vi "Display Fonts Manager.vi"(4 "Error In":errorcluster) -> (0 "Error Out":errorcluster)   [LabVIEW 2020, in "Display Properties Manager.lvlib"]
uses:
  Display Properties Manager.lvlib
  Display Properties.lvclass
  Config Data/Config Data.lvclass
  toolbox/Error Reporting and Storage/Error Reporting and Storage.lvlib
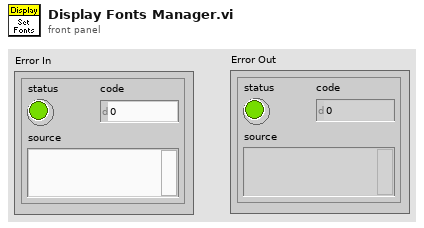
[diagram p1: front panel]
types:
  T1 = typedef "Display Properties Manager.lvlib/Font Parameters.ctl" = cluster{"Font Name":string, "Font Size":u32, "Component to Set":T2}
  T2 = typedef "Display Properties Manager.lvlib/Control Component to Set.ctl" = enum16{"Label", "Caption", "Contents"}
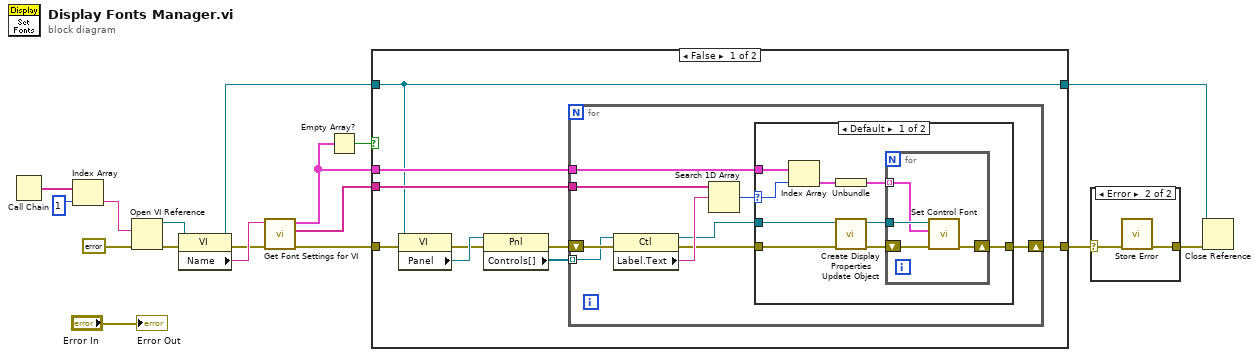
[diagram p0: block diagram]
diagram:
  n1 = Call Chain() -> (call chain=w12:string[])
  n2 = Index Array(array=w12, index=1) -> (element=w6:string)
  n3 = Open VI Reference(vi path=w6, error in (no error)=errorcluster {"status"=FALSE, "code"=0, "source"=""}) -> (vi reference=w7:refnum<vi>, error out=w10:errorcluster)  [unwired: 4 in]
  n4 = property class="VI"(reference=w7, error in=w10) -> (reference out=w8:refnum<vi>, error out=w9:errorcluster, "Name"=w13:string)
  n5 = call "Get Font Settings for VI.vi"("error in (no error)"=w9, "Name"=w13) -> ("error out"=w17:errorcluster, "Control Names"=w16:string[], "Font Parameters"=w15:cluster{T1[]}[])  [unwired: 3 in]
  n6 = Empty Array?(array=w15) -> (empty?=w14:bool)
  n7 = case shown="False" w14 {
    tunnel: w17 -> [w24 w51]
    tunnel: w8 -> [w18 w50]
    tunnel: [w19 w51] -> w2
    tunnel: w15 -> [w20 _]
    tunnel: w16 -> [w21 _]
    tunnel: [w18 w50] -> w5
    frame False {
      n8 = property class="VI"(reference=w18, error in=w24) -> (error out=w25:errorcluster, "Panel"=w26:refnum<vi>)  [unwired: 1 out]
      n9 = property class="Pnl"(reference=w26, error in=w25) -> (error out=w23:errorcluster, "Controls[]"=w22:refnum<vi>[])  [unwired: 1 out]
      n10 = for {
        shift-right: [w27] -> w19
        shift-left: w23 -> [w35]
        tunnel: w22 -> [w34] mode=indexing
        tunnel: w21 -> [w32]
        tunnel: w20 -> [w29]
        n11 = property class="Ctl"(reference=w34, error in=w35) -> (reference out=w28:refnum<vi>, error out=w30:errorcluster, "Label.Text"=w33:string)
        n12 = Search 1D Array(1D array=w32, element=w33) -> (index of element=w31:i32)  [unwired: 1 in]
        n13 = case shown="Default" w31 {
          selector: w31 -> [w44 _]
          tunnel: w30 -> [w42 w49]
          tunnel: [w38 w49] -> w27
          tunnel: w29 -> [w43 _]
          tunnel: w28 -> [w41 _]
          frame Default {
            n14 = Index Array(array=w43, index=w44) -> (element=w37:cluster{T1[]})
            n15 = Unbundle(w37) -> (w36:T1[])
            n16 = call "Create Display Properties Update Object.vi"("error in (no error)"=w42, "Control in"=w41) -> ("error out"=w39:errorcluster, "Font Settting out"=w40:refnum<class "Display Properties.lvclass">)  [unwired: 4 in]
            n17 = for {
              tunnel: w40 -> [w48]
              tunnel: w36 -> [w45] mode=indexing
              shift-right: [w46] -> w38
              shift-left: w39 -> [w47]
              n18 = call-dynamic "Set Control Font.vi"("Error In"=w47, "Font Parameters"=w45, "Font Settting in"=w48) -> ("Error Out"=w46:errorcluster)  [unwired: 3 in, 1 out]
            }
          }
          frame -1 {
          }
        }
      }
    }
    frame True {
    }
  }
  n19 = case shown="Error" w2 {
    selector: w2 -> [w52 w53]
    tunnel: [w52 w54] -> w1
    frame No Error {
    }
    frame Error {
      n20 = call "Store Error.vi"("error in (no error)"=w53) -> ("error out"=w54:errorcluster)  [unwired: 6 in]
    }
  }
  n21 = Close Reference(reference=w5, error in (no error)=w1) -> ()  [unwired: 1 out]
  "Error Out" <- "Error In"
